vi "OfflineColdStartMDrive.vi"(1 "Port Name":string) -> ()   [LabVIEW 2010]
panel:
  out "RepliesFromNewlySetupDrive":string[](array[string])
  in  "Address ToAssign":u8=1 min=1 max=9 step=1
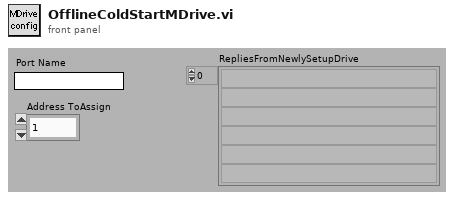
[diagram p1: front panel]
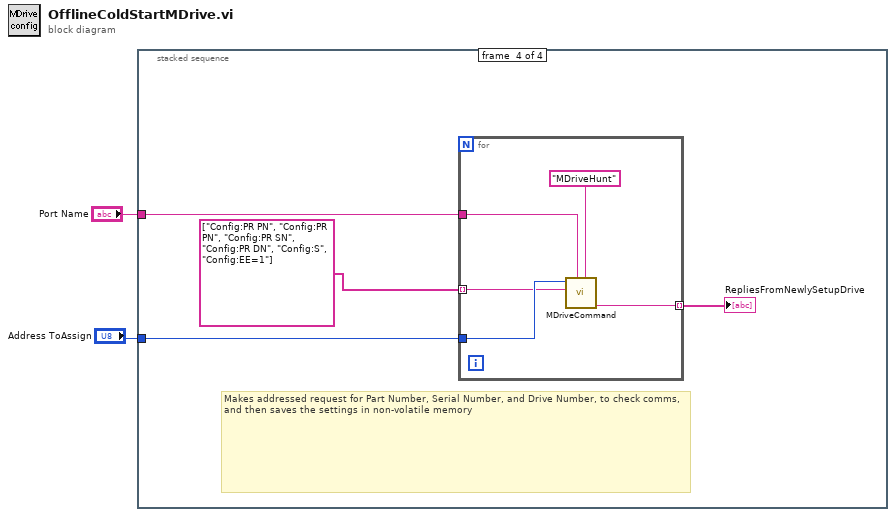
[diagram p0: block diagram]
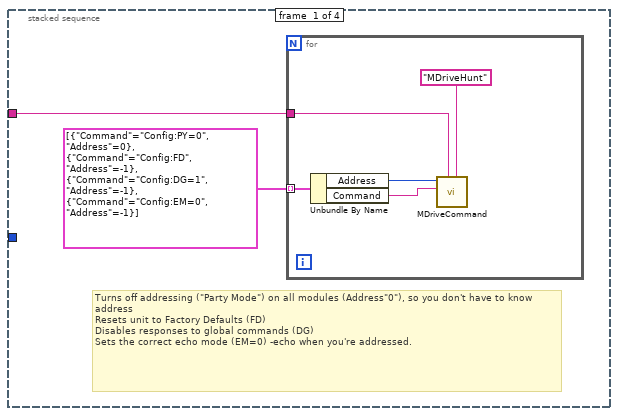
[diagram p2: hidden frame]
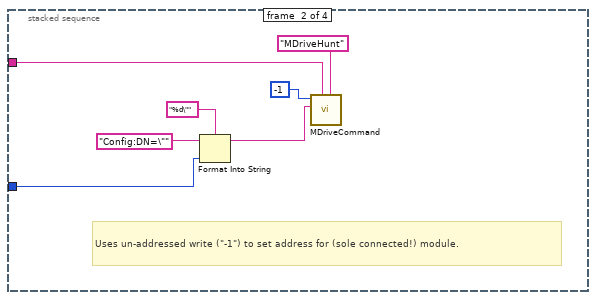
[diagram p3: hidden frame]
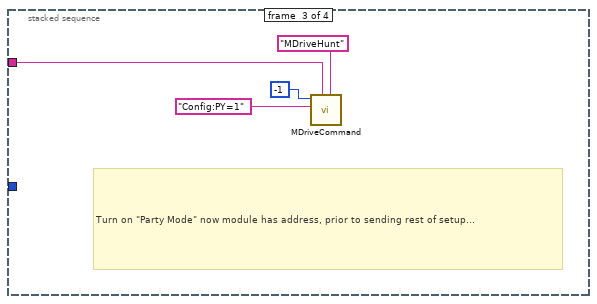
[diagram p4: hidden frame]
diagram:
  n1 = stacked-sequence {
    tunnel: "Port Name" -> [w4 w16 w20 w24]
    tunnel: "Address ToAssign" -> [_ w10 _ w22]
    frame #0 {
      # "Turns off addressing (\"Party Mode\") on all modules (Address\"0\"), so you don't have to know address\nResets unit to Factory Defaults (FD)\nDisables responses to global commands (DG)\nSets the correct echo mode (EM=0) -echo when you're addressed."
      n2 = for {
        tunnel: w4 -> [w9]
        tunnel: cluster{"Command":string, "Address":i8}[] [{"Command"="Config:PY=0", "Address"=0}, {"Command"="Config:FD", "Address"=-1}, {"Command"="Config:DG=1", "Address"=-1}, {"Command"="Config:EM=0", "Address"=-1}] -> [w7] mode=indexing
        n3 = Unbundle By Name(w7) -> ("Address"=w6:i8, "Command"=w5:string)
        n4 = call "MDriveCommand.vi"("Channel Name"="MDriveHunt", "Port Name"=w9, "MDriveCommand"=w5, "Address"=w6) -> ()  [unwired: 1 in, 6 out]
      }
    }
    frame #1 {
      # "Uses un-addressed write (\"-1\") to set address for (sole connected!) module."
      n5 = Format Into String(format string="%d\"", initial string="Config:DN=\"" ("string"), w10) -> (resulting string=w11:string)  [unwired: 1 in, 1 out]
      n6 = call "MDriveCommand.vi"("Channel Name"="MDriveHunt", "Port Name"=w16, "MDriveCommand"=w11, "Address"=i8 -1) -> ()  [unwired: 1 in, 6 out]
    }
    frame #2 {
      # "Turn on \"Party Mode\" now module has address, prior to sending rest of setup..."
      n7 = call "MDriveCommand.vi"("Channel Name"="MDriveHunt", "Port Name"=w20, "MDriveCommand"="Config:PY=1" ("string"), "Address"=i8 -1) -> ()  [unwired: 1 in, 6 out]
    }
    frame #3 {
      # "Makes addressed request for Part Number, Serial Number, and Drive Number, to check comms, and then saves the settings in non-volatile memory"
      n8 = for {
        tunnel: w24 -> [w29]
        tunnel: string[] ["Config:PR PN", "Config:PR PN", "Config:PR SN", "Config:PR DN", "Config:S", "Config:EE=1"] -> [w26] mode=indexing
        tunnel: w22 -> [w27]
        tunnel: [w25] -> w21 mode=indexing
        n9 = call "MDriveCommand.vi"("Channel Name"="MDriveHunt", "Port Name"=w29, "MDriveCommand"=w26, "Address"=w27) -> ("String Reply"=w25:string)  [unwired: 1 in, 5 out]
      }
      "RepliesFromNewlySetupDrive" <- w21
    }
  }
